vi "LDT Parse XML Timestamp.vi"(8 "error in":errorcluster, 11 "Time":string="2020-09-14T20:44:15.228+00:00") -> (0 "error out":errorcluster, 3 "Tempstamp":timestamp format="%<%H:%M:%S%3u\n%Y/%m/%d>T")   [LabVIEW 2022 SP3, in "LDT Telescope.lvclass"]
uses:
  LDT Telescope.lvclass
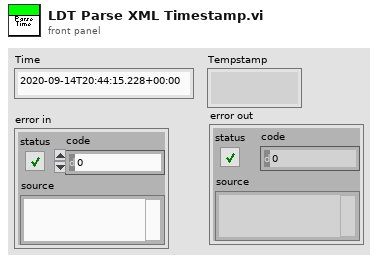
[diagram p1: front panel]
types:
  T1 = typedef "LVDateTimeRec.ctl" = cluster{"fractional second":dbl, "second":i32, "minute":i32, "hour":i32, "day of month":i32, "month":i32, "year":i32, "day of week":i32, "day of year":i32, "DST":i32}
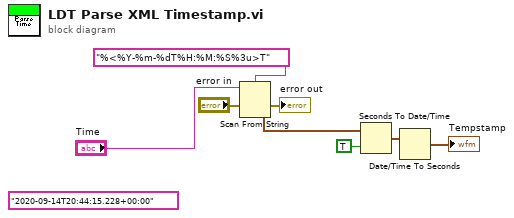
[diagram p0: block diagram]
diagram:
  (unwired) "2020-09-14T20:44:15.228+00:00" ("Time")
  n1 = Scan From String(format string="%<%Y-%m-%dT%H:%M:%S%3u>T", input string="Time", error in="error in") -> (error out=→"error out":errorcluster, output 1=w2:timestamp)  [unwired: 2 in, 2 out]
  n2 = Seconds To Date/Time(time stamp (now)=w2, to UTC (F)=TRUE) -> (date time rec=w4:T1)
  n3 = Date/Time To Seconds(2:w4) -> (0:→"Tempstamp":timestamp)  [unwired: 1 in]
